vi "Defer Panel Updates Wrapper.vi"(8 "error in":errorcluster, 10 "Defer Updates":bool, 11 "VI":refnum<vi>) -> (0 "error out":errorcluster)   [LabVIEW 2020]
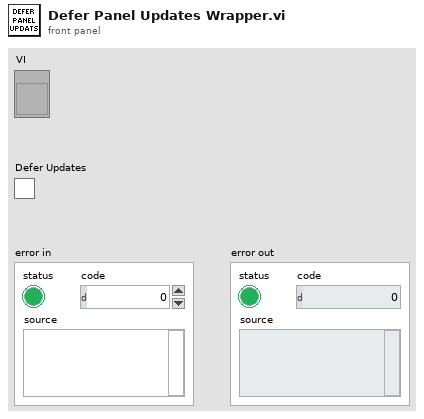
[diagram p1: front panel]
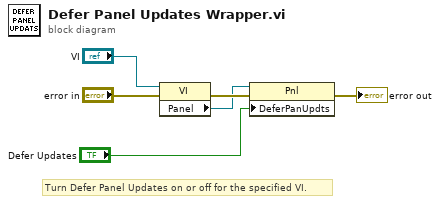
[diagram p0: block diagram]
diagram:
  # "Turn Defer Panel Updates on or off for the specified VI."
  n1 = property class="VI"(reference="VI", error in="error in") -> (error out=w5:errorcluster, "Panel"=w2:refnum<vi>)  [unwired: 1 out]
  n2 = property class="Pnl"(reference=w2, error in=w5, "DeferPanUpdts"="Defer Updates") -> (error out=→"error out":errorcluster)  [unwired: 1 out]
